vi "PH_Stepmotor_BaseClass.ProcEvents.vi"(0 "i ref in":refnum<vi>, 5 "error in":errorcluster) -> (14 "i ref out":refnum<vi>, 19 "error out":errorcluster)   [LabVIEW 2014, in "PH_Stepmotor_BaseClass.lvlib"]
doc: "This method is used during the 1st frame of the process object to define the events the object will listen to. Add your own events here."
uses:
  PH_Stepmotor_BaseClass.lvlib
  CS_Core/BaseProcess/BaseProcess.event definition.ctl
  CS_Core/CAEObj/CAEObj.event definition.ctl
  CS_Core/BaseProcess/BaseProcess.descriptor string definition.ctl
  CS_Core/BaseProcess/BaseProcess.lvlib
  CS_Core/CAEObj/CAEObj.lvlib
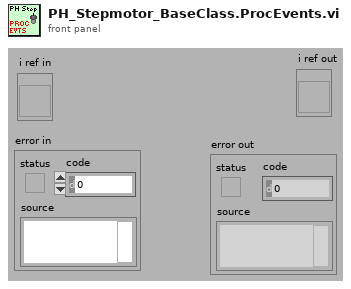
[diagram p1: front panel]
types:
  T1 = typedef "BaseProcess.lvlib/BaseProcess.event definition.ctl" = cluster{"CAEEvtDef":T2, "Data Descriptor":T3}
  T2 = typedef "CAEObj.lvlib/CAEObj.event definition.ctl" = cluster{"URL":string, "enable":bool, "ignoreResID":bool}
  T3 = typedef "BaseProcess.lvlib/BaseProcess.descriptor string definition.ctl" = string
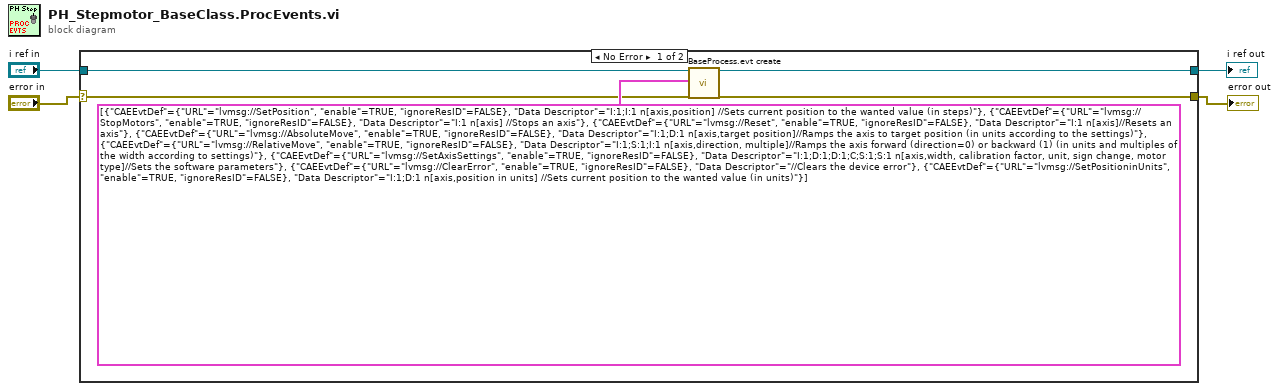
[diagram p0: block diagram]
diagram:
  n1 = case shown="No Error" "error in" {
    selector: "error in" -> [w5 w11]
    tunnel: "i ref in" -> [w6 w10]
    tunnel: [w9 w10] -> w3
    tunnel: [w8 w11] -> w2
    frame No Error {
      n2 = call "BaseProcess.evt create.vi"("i ref in"=w6, "newEvents"=T1[] [{"CAEEvtDef"={"URL"="lvmsg://SetPosition", "enable"=TRUE, "ignoreResID"=FALSE}, "Data Descriptor"="I:1;I:1 n[axis,position] //Sets current position to the wanted value (in steps)"}, {"CAEEvtDef"={"URL"="lvmsg://StopMotors", "enable"=TRUE, "ignoreResID"=FALSE}, "Data Descriptor"="I:1 n[axis] //Stops an axis"}, {"CAEEvtDef"={"URL"="lvmsg://Reset", "enable"=TRUE, "ignoreResID"=FALSE}, "Data Descriptor"="I:1 n[axis]//Resets an axis"}, {"CAEEvtDef"={"URL"="lvmsg://AbsoluteMove", "enable"=TRUE, "ignoreResID"=FALSE}, "Data Descriptor"="I:1;D:1 n[axis,target position]//Ramps the axis to target position (in units according to the settings)"}, {"CAEEvtDef"={"URL"="lvmsg://RelativeMove", "enable"=TRUE, "ignoreResID"=FALSE}, "Data Descriptor"="I:1;S:1;I:1 n[axis,direction, multiple]//Ramps the axis forward (direction=0) or backward (1) (in units and multiples of the width according to settings)"}, {"CAEEvtDef"={"URL"="lvmsg://SetAxisSettings", "enable"=TRUE, "ignoreResID"=FALSE}, "Data Descriptor"="I:1;D:1;D:1;C;S:1;S:1 n[axis,width, calibration factor, unit, sign change, motor type]//Sets the software parameters"}, {"CAEEvtDef"={"URL"="lvmsg://ClearError", "enable"=TRUE, "ignoreResID"=FALSE}, "Data Descriptor"="//Clears the device error"}, {"CAEEvtDef"={"URL"="lvmsg://SetPositioninUnits", "enable"=TRUE, "ignoreResID"=FALSE}, "Data Descriptor"="I:1;D:1 n[axis,position in units] //Sets current position to the wanted value (in units)"}] ("appended array"), "error in (no error)"=w5) -> ("i ref out"=w9:refnum<vi>, "error out"=w8:errorcluster)  [unwired: 13 in, 2 out]
    }
    frame Error {
    }
  }
  "i ref out" <- w3
  "error out" <- w2
